vi "Read WebSocket Service Enqueuer.vi"(8 "error in (no error)":errorcluster, 11 "WS Test Server in":refnum<class "WS Server Subscriber.lvclass">) -> (0 "error out":errorcluster, 2 "Actor Framework:Message Enqueuer":refnum<class "Message Enqueuer.lvclass">, 3 "WS Test Server out":refnum<class "WS Server Subscriber.lvclass">)   [LabVIEW 2021, in "Echo Broadcast With Server Manager.lvlib" / "WS Server Subscriber.lvclass"]
uses:
  WS Server Subscriber.lvclass
  <vilib>/ActorFramework/Message Enqueuer/Message Enqueuer.lvclass
  WS Server Subscriber.lvclass/WS Server Subscriber.ctl
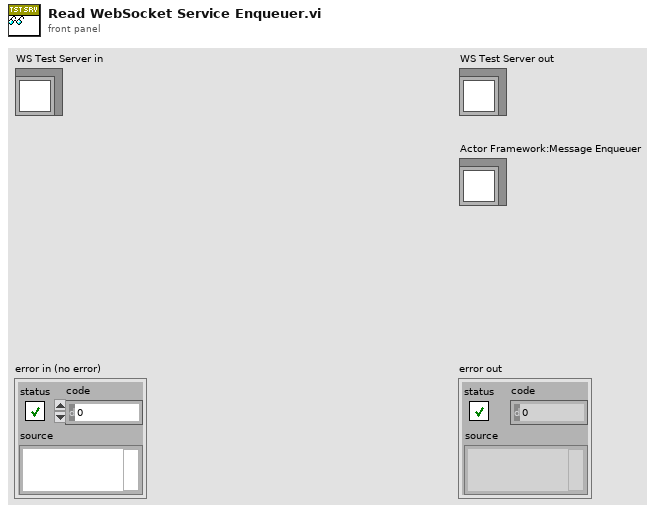
[diagram p1: front panel]
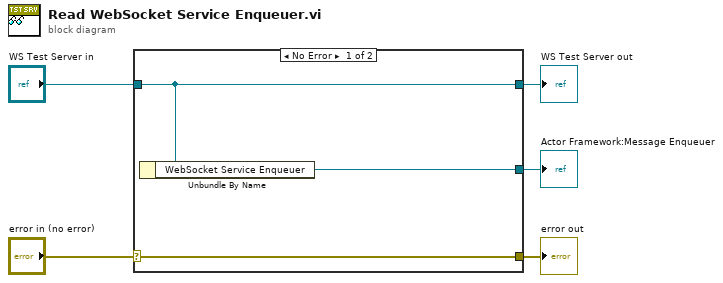
[diagram p0: block diagram]
diagram:
  n1 = case shown="No Error" "error in (no error)" {
    selector: "error in (no error)" -> [w8 w9]
    tunnel: [w8 w9] -> w4
    tunnel: [w7 w10] -> w2
    tunnel: "WS Test Server in" -> [w7 w10]
    tunnel: [w6 _] -> w1
    frame No Error {
      n2 = Unbundle By Name(w7) -> ("WebSocket Service Enqueuer"=w6:refnum<class "Message Enqueuer.lvclass">)
    }
    frame Error {
    }
  }
  "error out" <- w4
  "WS Test Server out" <- w2
  "Actor Framework:Message Enqueuer" <- w1
